vi "Draw.vi"(8 "error in (no error)":errorcluster, 9 "disable contained items?":bool, 10 "IB_Tree":refnum<class "IB_Tree.lvclass">, 11 "IB_TreeCtrFileItem in":refnum<class "IB_Tree_Item_Source_Contained_File.lvclass">) -> (0 "error out":errorcluster, 3 "IB_TreeCtrFileItem out":refnum<class "IB_Tree_Item_Source_Contained_File.lvclass">)   [LabVIEW 2020, in "IB_Tree_Item_Source_Contained_File.lvclass"]
uses:
  <vilib>/AppBuilder/IB_Classes/Tree_Item_Source_Contained_File/IB_Tree_Item_Source_Contained_File.lvclass
  <vilib>/AppBuilder/IB_Classes/Tree_Item_Source_Contained_File/IB_Tree_Item_Source_Contained_File.lvclass/IB_Tree_Item_Source_Contained_File.ctl
  <vilib>/AppBuilder/IB_Classes/Tree_Item_Virtual_Folder/IB_Tree_Item_Virtual_Folder.lvclass
  <vilib>/AppBuilder/IB_Classes/Tree_Item_Source_File/IB_Tree_Item_Source_File.lvclass
  <vilib>/AppBuilder/IB_Classes/Tree/IB_Tree.lvclass
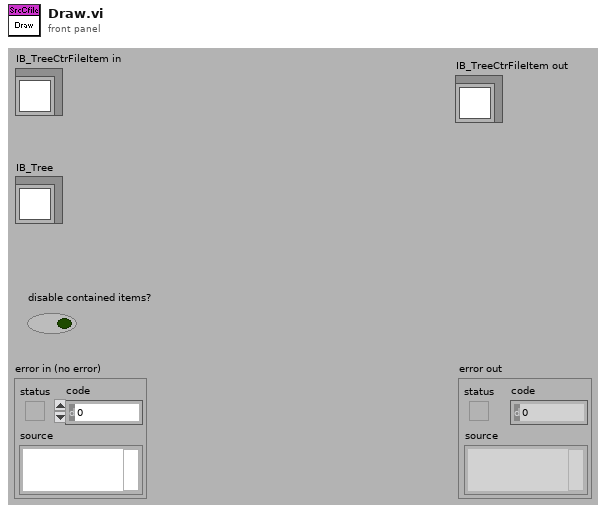
[diagram p1: front panel]
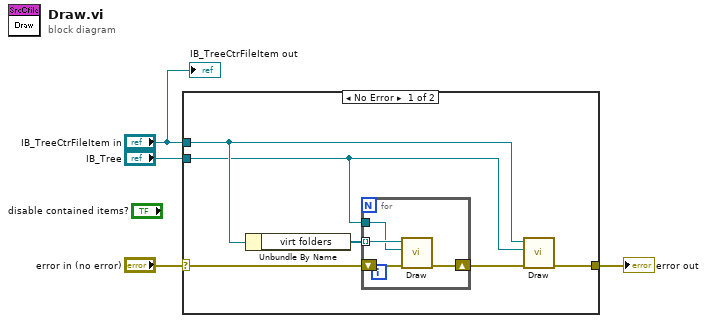
[diagram p0: block diagram]
diagram:
  n1 = case shown="No Error" "error in (no error)" {
    selector: "error in (no error)" -> [w5 w15]
    tunnel: [w10 w15] -> w4
    tunnel: "IB_TreeCtrFileItem in" -> [w9 _]
    tunnel: "IB_Tree" -> [w7 _]
    frame No Error {
      n2 = Unbundle By Name(w9) -> ("virt folders"=w8:refnum<class "IB_Tree_Item_Virtual_Folder.lvclass">[])
      n3 = for {
        tunnel: w8 -> [w14] mode=indexing
        tunnel: w7 -> [w13]
        shift-right: [w11] -> w6
        shift-left: w5 -> [w12]
        n4 = call-dynamic "Draw.vi"("error in (no error)"=w12, "IB_Tree"=w13, "IB_TreeItem in"=w14) -> ("error out"=w11:errorcluster)  [unwired: 1 in, 7 out]
      }
      n5 = call-parent "Draw.vi"("error in (no error)"=w6, "IB_Tree"=w7, "IB_TreeItem in"=w9) -> ("error out"=w10:errorcluster)  [unwired: 1 in, 7 out]
    }
    frame Error {
    }
  }
  "error out" <- w4
  "IB_TreeCtrFileItem out" <- "IB_TreeCtrFileItem in"
